vi "UI_Control_System.vi"() -> ()   [LabVIEW 2014]
uses:
  <vilib>/Platform/TimedLoop/XDataNode/timing_clust.ctl
  <vilib>/Platform/TimedLoop/XDataNode/nitl_modes.ctl
  <vilib>/Platform/TimedLoop/XDataNode/wakeup.ctl
  Terminal-Global-SetValues.vi
  <vilib>/Platform/TimedLoop/XDataNode/XDataNode.xnode
  <vilib>/Platform/TimedLoop/XDataNode/XDNodeRunTimeDep.lvlib
panel:
  out "载荷谱修改":bool=TRUE
  in  "载荷谱修改":bool
  in  "停止":bool caption="启动"
  in  "系统执行状态":i32(listbox)
  out "右侧Y位移":sgl[](graph)
  out "右侧X位移":sgl[](graph)
  out "左侧Y位移":sgl[](graph)
  out "左侧X位移":sgl[](graph)
  in  "加载单元查看详细":bool caption="加载单元"
  in  "主轴监测单元查看详细":bool caption="加载单元"
  in  "试验单元查看详细":bool caption="加载单元"
  in  "陪试单元查看详细":bool caption="加载单元"
  in  "实验进度":dbl(slide) scale=0.0..100.0 scale format="%#_g%%"
  out "Data":string caption="当前时间："
  out "轴向位移幅度图":sgl[](graph)
  out "右侧轴心轨迹图":cluster{"电涡流3":sgl[], "电涡流4":sgl[]}(graph)
  out "左侧轴心轨迹图":cluster{"电涡流1":sgl[], "电涡流2":sgl[]}(graph)
  out "转速":sgl
  out "出油温度2":dbl
  out "出油温度1":dbl
  out "试验单元出油温度":dbl
  out "轴承外圈温度":dbl
  out "试验单元摩擦力矩":dbl
  out "声发射频谱图":sgl[](graph)
  out "声发射时间曲线":sgl[](graph)
  out "外壳振动频谱图":dbl(graph)
  out "外壳振动时间曲线":cluster{"加速度2":sgl[]}[](graph)
  out "轴向液压缸加载压力":dbl
  out "径向液压缸加载压力":dbl
  # "轴承测控系统"
  # "检测参数区域"
  # "主轴监测单元"
  # "加载单元"
  # "陪试单元"
  # "实验单元"
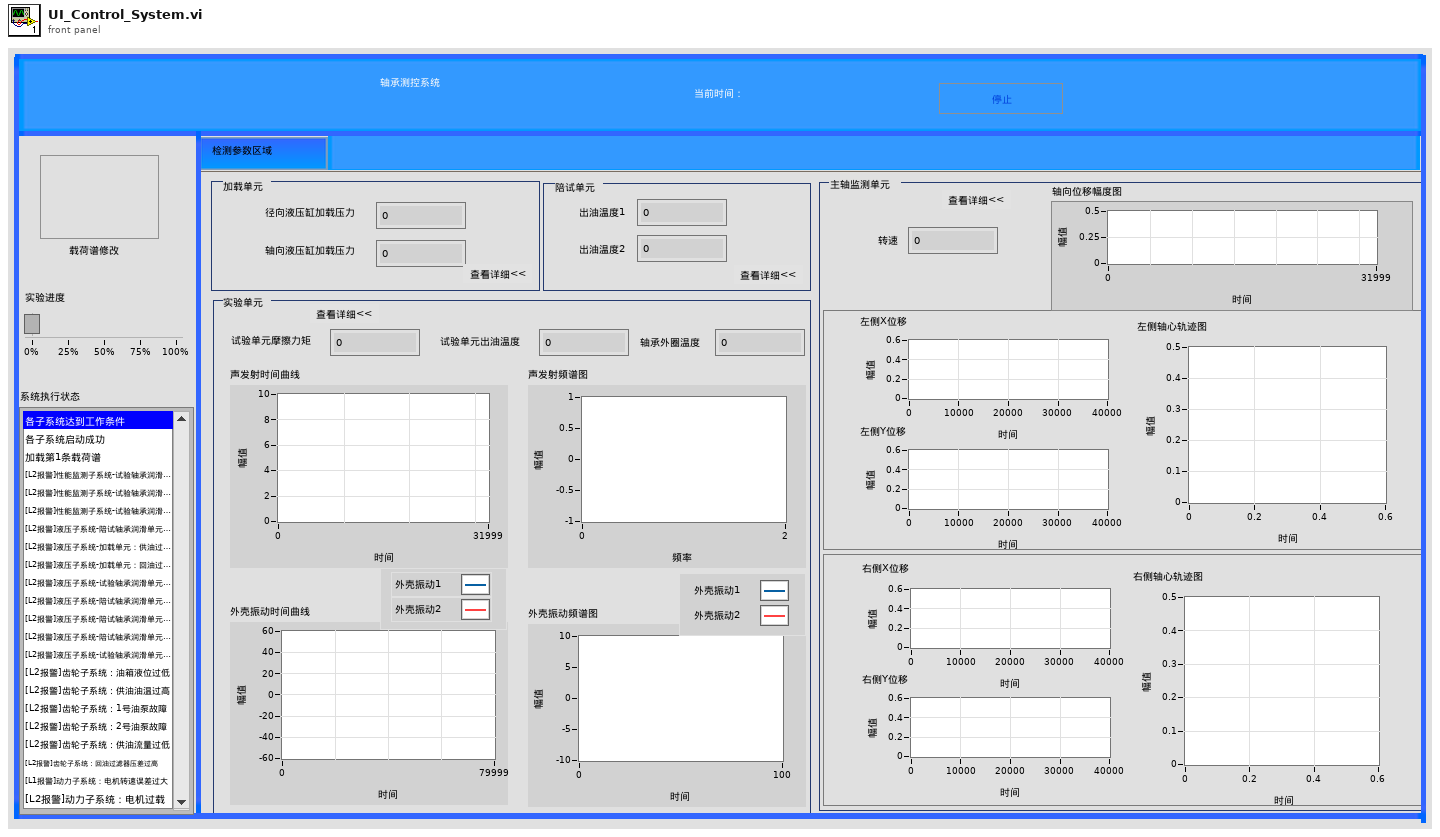
[diagram p1: front panel]
types:
  T1 = typedef "XDNodeRunTimeDep.lvlib/timing_clust.ctl" = cluster{"Expected End [f-1]":u64, "Actual End [f-1]":u64, "Finished Late? [f-1]":bool, "Expected End [i-1]":u64, "Actual End [i-1]":u64, "Finished Late? [i-1]":bool, "Expected Start [i]":u64, "Actual Start [i]":u64, "Expected Start [f]":u64, "Actual Start [f]":u64, "Source Name":string, "Structure Name":string, "Period":i64, "Deadline":i64, "Offset":i64, "Start":i64, "Priority":i32, "Timeout":i32, "Mode":T2, "Wakeup Reason":T3, "Error":errorcluster, "Source Type":string, "Secondary Source Type":string, "Global End Time":u64, "Global Start Time":u64, "Frame Duration":u64, "Iteration Duration":u64, "Assigned CPU":i32, "I/O Scan Engine Mode":u32}
  T2 = typedef "XDNodeRunTimeDep.lvlib/nitl_modes.ctl" = enum32{"No Change", "Process missed periods, maintain original phase", "Discard missed periods, maintain original phase", "Process missed periods, ignore original phase", "Discard missed periods, ignore original phase"}
  T3 = typedef "XDNodeRunTimeDep.lvlib/wakeup.ctl" = enum32{"Normal", "Aborted", "Asynchronous wakeup", "Timing source error", "Timed loop error", "Timeout"}
  T4 = cluster{"润滑油流量":u16, "油箱润滑油液位":u16, "油箱温度":u16, "冷却装置工作状态":u16, "供油压力":u16, "过滤器压差":u16, "油箱液位":u16, "供油油温":u16, "齿轮箱轴承温度":u16, "齿轮箱高速端输出转速":u16, "齿轮子系统状态字":cluster{"加热装置异常报警":bool, "冷却装置异常报警":bool, "油箱液位过低报警":bool, "供油油温过高报警":bool, "循环回路过滤器压差过高报警":bool, "1号油泵故障报警":bool, "2号油泵故障报警":bool, "供油压力过低报警":bool, "供油流量过低报警":bool, "轴承温度异常报警":bool, "油箱液位过高报警":bool, "回油过滤器压差过高报警":bool, "供油过滤器压差过高报警":bool}}
  T5 = cluster{"径向油缸加载压力":u16, "轴向油缸加载压力":u16, "油箱1油液温度":u16, "润滑油温度":u16, "油箱2油液温度":u16, "试验轴承供油压力":u16, "试验轴承供油流量":u16, "陪试轴承供油流量":u16, "陪试轴承供油压力":u16, "陪试轴承供油温度":u16, "液压子系统状态字":cluster{"加载单元":cluster{"供油过滤器堵塞报警":bool, "回油过滤器堵塞报警":bool, "液位过高报警":bool, "液位过低报警":bool}, "试验轴承单元":cluster{"加热装置异常报警":bool, "油箱1液位过高报警":bool, "油箱1液位过低报警":bool, "油箱2液位过高报警":bool, "油箱2液位过低报警":bool, "供油过滤器堵塞报警":bool, "循环回路过滤器堵塞报警":bool, "回油过滤器堵塞报警":bool}, "陪试轴承单元":cluster{"供油过滤器1堵塞报警":bool, "供油过滤器2堵塞报警":bool, "回油过滤器堵塞报警":bool, "油箱液位过高报警":bool, "油箱液位过低报警":bool}}}
  T6 = cluster{"时间":timestamp, "陪试轴承润滑单元出油温度1":sgl[], "陪试轴承润滑单元出油温度2":sgl[], "轴承外圈温度":sgl[], "出油温度":sgl[], "摩擦力1":sgl[], "摩擦力2":sgl[], "径向油缸力":sgl[], "轴向油缸力":sgl[], "转速":sgl[]}
  T7 = cluster{"时间":timestamp, "声发射":sgl[], "电涡流1":sgl[], "电涡流2":sgl[], "电涡流3":sgl[], "电涡流4":sgl[], "电涡流5":sgl[], "加速度1":sgl[], "加速度2":sgl[]}
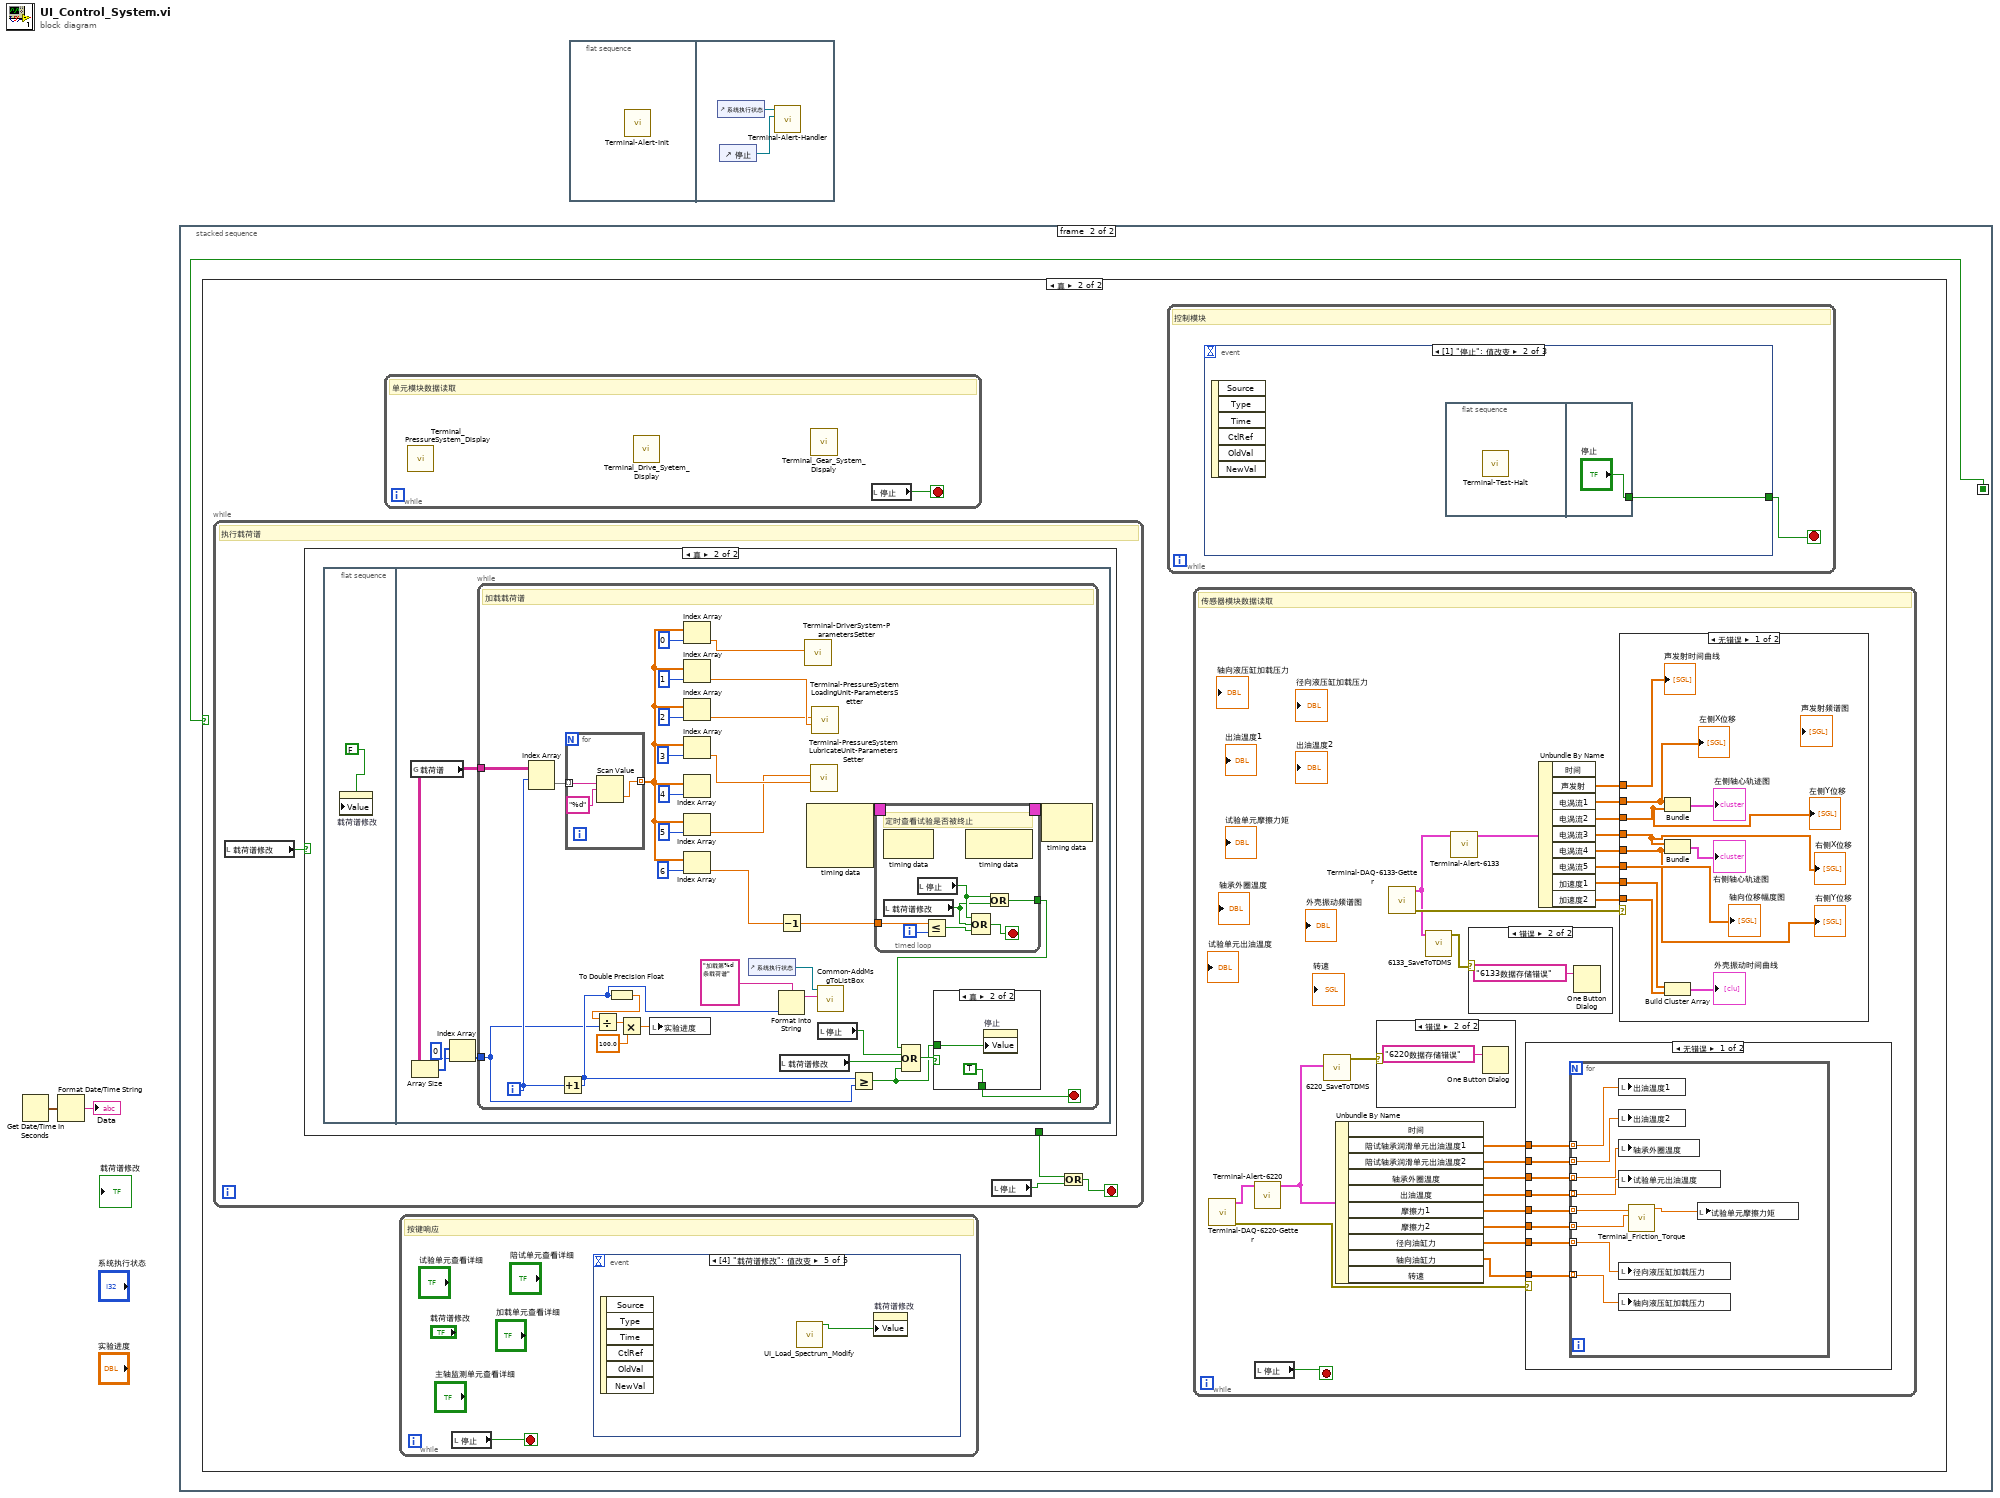
[diagram p0: block diagram]
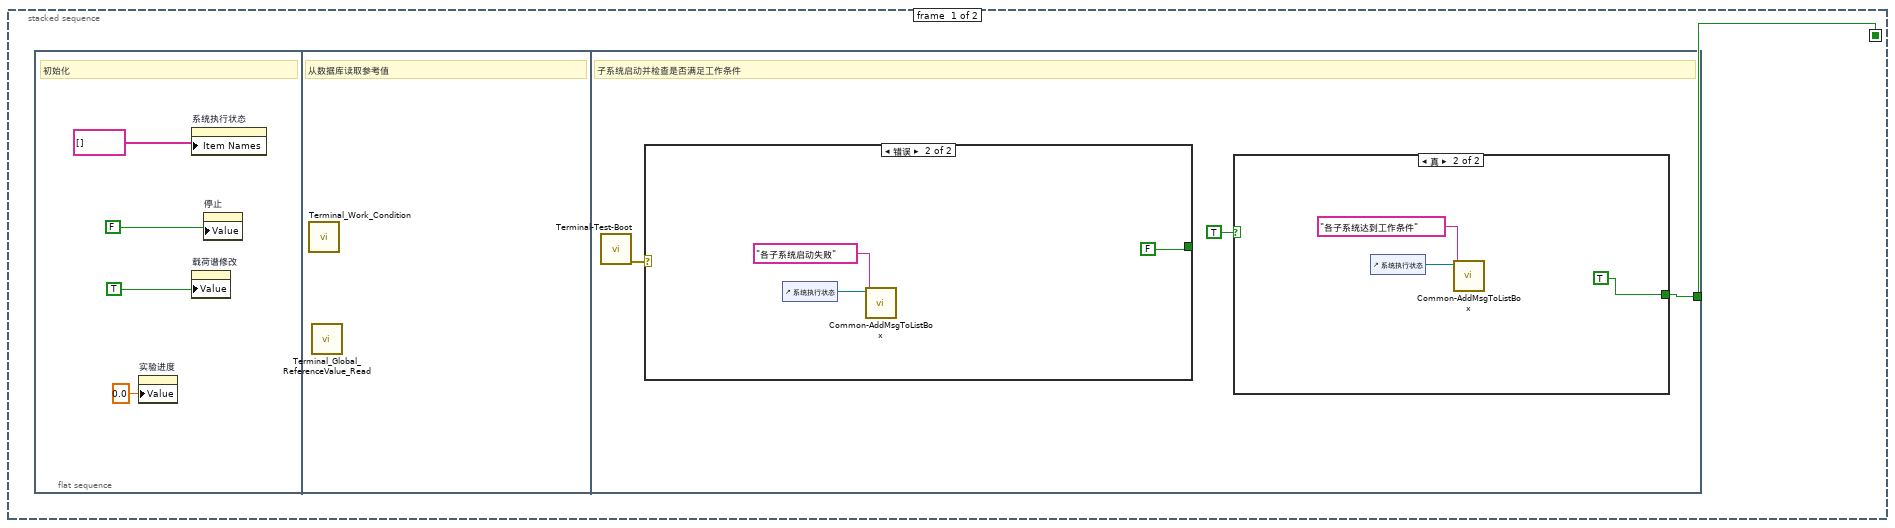
[diagram p2: hidden frame]
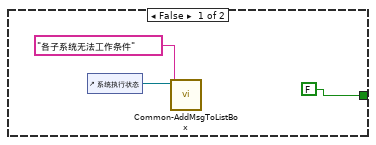
[diagram p3: hidden frame]
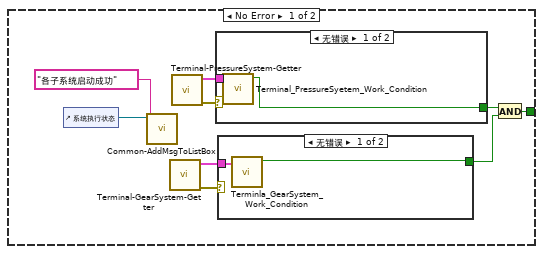
[diagram p4: hidden frame]
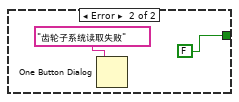
[diagram p5: hidden frame]
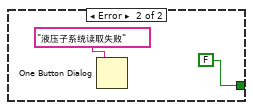
[diagram p6: hidden frame]
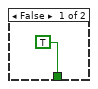
[diagram p8: hidden frame]
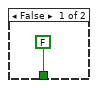
[diagram p9: hidden frame]
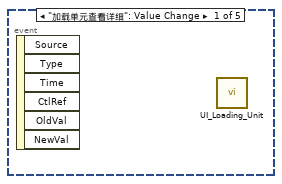
[diagram p10: hidden frame]
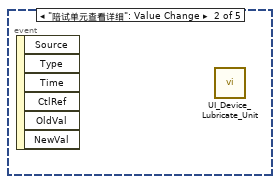
[diagram p11: hidden frame]
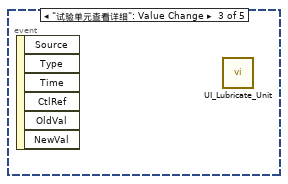
[diagram p12: hidden frame]
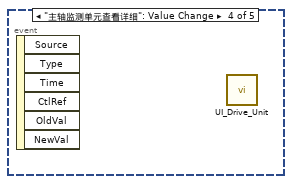
[diagram p13: hidden frame]
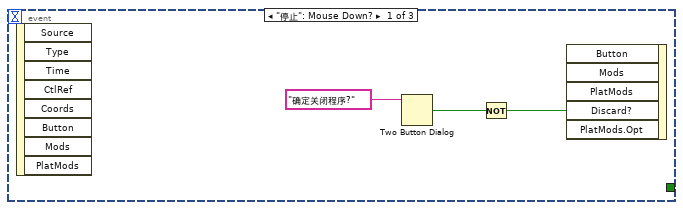
[diagram p18: hidden frame]
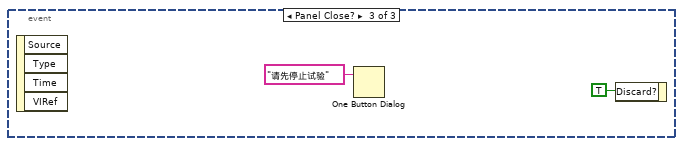
[diagram p19: hidden frame]
diagram:
  n1 = Get Date/Time In Seconds() -> (seconds since 1Jan1904=w1:timestamp)
  n2 = Format Date/Time String(seconds (now)=w1) -> (date/time string=→"Data":string)  [unwired: 2 in]
  n3 = stacked-sequence {
    seq-local: [w3 _] -> [_ w37]
    frame #0 {
      n4 = flat-sequence {
        tunnel: [w8] -> w3
        frame #0 {
          # "初始化"
          n5 = property on="实验进度" class="Slide (严格)"("Value"=0.0 ("实验进度")) -> ()  [unwired: 2 in, 2 out]
          n6 = property on="系统执行状态" class="LstBox (严格)"("Item Names"=string[] [] ("项名")) -> ()  [unwired: 2 in, 2 out]
          n7 = property on="载荷谱修改" class="Bool (严格)"("Value"=TRUE) -> ()  [unwired: 2 in, 2 out]
          n8 = property on="停止" class="Bool (严格)"("Value"=FALSE) -> ()  [unwired: 2 in, 2 out]
        }
        frame #1 {
          # "从数据库读取参考值"
          n9 = call "Terminal_Work_Condition.vi"() -> ()  [unwired: 12 in]
          n10 = call "Terminal_Global_ReferenceValue_Read.vi"() -> ()  [unwired: 12 in]
        }
        frame #2 {
          # "子系统启动并检查是否满足工作条件"
          n11 = call "Terminal-Test-Boot.vi"() -> ("error out"=w10:errorcluster)  [unwired: 11 in]
          n12 = case shown="错误" w10 {
            tunnel: [w21 FALSE] -> _
            frame No Error {
              n13 = control-ref of="系统执行状态"() -> (w17:refnum<vi>)
              n14 = call "Common-AddMsgToListBox.vi"("字符串"="各子系统启动成功", "列表框"=w17) -> ()  [unwired: 10 in]
              n15 = call "Terminal-GearSystem-Getter.vi"() -> ("error out"=w19:errorcluster, "设备信息"=w24:T4)  [unwired: 9 in, 1 out]
              n16 = call "Terminal-PressureSystem-Getter.vi"() -> ("error out"=w20:errorcluster, "设备信息"=w25:T5)  [unwired: 9 in, 1 out]
              n17 = case shown="无错误" w20 {
                tunnel: w25 -> [w31 _]
                tunnel: [w30 FALSE] -> w23
                frame No Error {
                  n18 = call "Terminal_PressureSyetem_Work_Condition.vi"("液压子系统监测参数"=w31) -> ("达到工作条件"=w30:bool)  [unwired: 10 in]
                }
                frame Error {
                  n19 = One Button Dialog(message="液压子系统读取失败" ("消息")) -> ()  [unwired: 1 in, 1 out]
                }
              }
              n20 = case shown="无错误" w19 {
                tunnel: w24 -> [w27 _]
                tunnel: [w26 FALSE] -> w22
                frame No Error {
                  n21 = call "Terminla_GearSystem_Work_Condition.vi"("齿轮子系统监测参数"=w27) -> ("达到工作条件"=w26:bool)  [unwired: 10 in]
                }
                frame Error {
                  n22 = One Button Dialog(message="齿轮子系统读取失败" ("消息")) -> ()  [unwired: 1 in, 1 out]
                }
              }
              n23 = And(x=w23, y=w22) -> (x .and. y?=w21:bool)
            }
            frame Error {
              n24 = control-ref of="系统执行状态"() -> (w34:refnum<vi>)
              n25 = call "Common-AddMsgToListBox.vi"("字符串"="各子系统启动失败", "列表框"=w34) -> ()  [unwired: 10 in]
            }
          }
          n26 = case shown="真" TRUE {
            tunnel: [FALSE TRUE] -> w8
            frame False {
              n27 = control-ref of="系统执行状态"() -> (w13:refnum<vi>)
              n28 = call "Common-AddMsgToListBox.vi"("字符串"="各子系统无法工作条件", "列表框"=w13) -> ()  [unwired: 10 in]
            }
            frame True {
              n29 = control-ref of="系统执行状态"() -> (w16:refnum<vi>)
              n30 = call "Common-AddMsgToListBox.vi"("字符串"="各子系统达到工作条件", "列表框"=w16) -> ()  [unwired: 10 in]
            }
          }
        }
      }
    }
    frame #1 {
      n31 = case shown="真" w37 {
        frame False {
        }
        frame True {
          n32 = while {
            stop <- w39 stop-if-true
            # "执行载荷谱"
            n33 = local read "载荷谱修改"() -> (w41:bool)
            n34 = case shown="真" w41 {
              tunnel: [TRUE _] -> w38
              frame False {
              }
              frame True {
                n35 = flat-sequence {
                  frame #0 {
                    n36 = property on="载荷谱修改" class="Bool (严格)"("Value"=FALSE) -> ()  [unwired: 2 in, 2 out]
                  }
                  frame #1 {
                    n37 = global read "Terminal-Global-SetValues.vi" "载荷谱"() -> (w47:string[][])
                    n38 = Array Size(array=w47) -> (size(s)=w46:i32[])
                    n39 = Index Array(array=w46, index=0 ("索引")) -> (element=w45:i32)
                    n40 = while {
                      tunnel: w47 -> [w66]
                      tunnel: w45 -> [w57]
                      i -> [w65]
                      stop <- w58 stop-if-true
                      # "加载载荷谱"
                      n41 = Index Array(array=w66, index (row)=w65) -> (element=w82:string[])  [unwired: 1 in]
                      n42 = Increment(x=w65) -> (x+1=w59:i32)
                      n43 = for {
                        tunnel: w82 -> [w99] mode=indexing
                        tunnel: [w97] -> w81 mode=indexing
                        n44 = Scan Value(string=w99, format string="%d" ("格式字符串")) -> (value=w97:dbl)  [unwired: 1 in, 1 out]
                      }
                      n45 = To Double Precision Float(number=w59) -> (double precision float=w64:dbl)
                      n46 = Divide(x=w64, y=w57) -> (x/y=w62:dbl)
                      n47 = Multiply(x=w62, y=100.0) -> (x*y=w60:dbl)
                      n48 = local write "实验进度"(w60) -> ()
                      n49 = Index Array(array=w81, index=0 ("索引")) -> (element=w71:dbl)
                      n50 = Index Array(array=w81, index=1 ("索引")) -> (element=w70:dbl)
                      n51 = Index Array(array=w81, index=2 ("索引")) -> (element=w69:dbl)
                      n52 = Index Array(array=w81, index=3 ("索引")) -> (element=w68:dbl)
                      n53 = Index Array(array=w81, index=4 ("索引")) -> ()  [unwired: 1 out]
                      n54 = Index Array(array=w81, index=5 ("索引")) -> (element=w67:dbl)
                      n55 = Index Array(array=w81, index=6 ("索引")) -> (element=w54:dbl)
                      n56 = control-ref of="系统执行状态"() -> (w73:refnum<vi>)
                      n57 = Decrement(x=w54) -> (x-1=w53:dbl)
                      n58 = Format Into String(format string="加载第%d条载荷谱" ("字符串"), w59) -> (resulting string=w72:string)  [unwired: 2 in, 1 out]
                      n59 = local read "载荷谱修改"() -> (w50:bool)
                      n60 = call "Terminal-DriverSystem-ParametersSetter.vi"("转速"=w71) -> ()  [unwired: 10 in, 1 out]
                      n61 = node-c288() -> (w56:T1)  [unwired: 3 in]
                      n62 = call "Terminal-PressureSystemLubricateUnit-ParametersSetter.vi"("供油润滑温度T"=w68, "供油流量L"=w67) -> ()  [unwired: 9 in, 1 out]
                      n63 = call "Terminal-PressureSystemLoadingUnit-ParametersSetter.vi"("轴向载荷F2"=w70, "径向载荷F1"=w69) -> ()  [unwired: 9 in, 1 out]
                      n64 = call "Common-AddMsgToListBox.vi"("字符串"=w72, "列表框"=w73) -> ()  [unwired: 10 in]
                      n65 = local read "停止"() -> (w51:bool)
                      n66 = Greater Or Equal?(x=w59, y=w57) -> (x >= y?=w49:bool)
                      n67 = timed-loop {
                        timing: w56 -> [_]
                        timing-out: [_] -> w55
                        tunnel: w53 -> [w89]
                        tunnel: [w83] -> w48
                        i -> [w88]
                        stop <- w87 stop-if-true
                        # "定时查看试验是否被终止"
                        n68 = node-c288() -> ()  [unwired: 1 in, 1 out]
                        n69 = local read "载荷谱修改"() -> (w84:bool)
                        n70 = local read "停止"() -> (w85:bool)
                        n71 = Less Or Equal?(x=w89, y=w88) -> (x <= y?=w86:bool)
                        n72 = node-c288() -> ()  [unwired: 1 in, 1 out]
                        n73 = Compound Arithmetic op=OR(w85, w84, w86) -> (w87:bool)
                        n74 = Or(x=w85, y=w84) -> (x .or. y?=w83:bool)
                      }
                      n75 = Compound Arithmetic op=OR(w48, w51, w50, w49) -> (w52:bool)
                      n76 = case shown="真" w52 {
                        tunnel: [FALSE ("停止") TRUE ("停止")] -> w58
                        tunnel: w49 -> [_ w95]
                        frame False {
                        }
                        frame True {
                          n77 = property on="停止" class="Bool (严格)"("Value"=w95) -> ()  [unwired: 2 in, 2 out]
                        }
                      }
                      n78 = node-c288(w55) -> ()  [unwired: 1 out]
                    }
                  }
                }
              }
            }
            n79 = local read "停止"() -> (w40:bool)
            n80 = Or(x=w38, y=w40) -> (x .or. y?=w39:bool)
          }
          n81 = while {
            stop <- w102 stop-if-true
            # "单元模块数据读取"
            n82 = call "Terminal_PressureSystem_Display.vi"() -> ()  [unwired: 12 in]
            n83 = call "Terminal_Drive_Syetem_Display.vi"() -> ()  [unwired: 12 in]
            n84 = call "Terminal_Gear_System_Dispaly.vi"() -> ()  [unwired: 12 in]
            n85 = local read "停止"() -> (w102:bool)
          }
          n86 = while {
            stop <- w100 stop-if-true
            # "按键响应"
            n87 = local read "停止"() -> (w100:bool)
            n88 = event shown="[4] \"载荷谱修改\": 值改变" {
              selector: _ -> [_ _ _ _ _]
              dyn-events: _ -> [_ _ _ _ _]
              timeout: _ -> [_ _ _ _ _]
              event "加载单元查看详细": Value Change {
                n89 = event-data() -> ()  [unwired: 1 in, 6 out]
                n90 = call "UI_Loading_Unit.vi"() -> ()  [unwired: 12 in]
              }
              event "陪试单元查看详细": Value Change {
                n91 = event-data() -> ()  [unwired: 1 in, 6 out]
                n92 = call "UI_Device_Lubricate_Unit.vi"() -> ()  [unwired: 12 in]
              }
              event "试验单元查看详细": Value Change {
                n93 = event-data() -> ()  [unwired: 1 in, 6 out]
                n94 = call "UI_Lubricate_Unit.vi"() -> ()  [unwired: 12 in]
              }
              event "主轴监测单元查看详细": Value Change {
                n95 = event-data() -> ()  [unwired: 1 in, 6 out]
                n96 = call "UI_Drive_Unit.vi"() -> ()  [unwired: 12 in]
              }
              event "载荷谱修改": Value Change {
                n97 = event-data() -> ()  [unwired: 1 in, 6 out]
                n98 = call "UI_Load_Spectrum_Modify.vi"() -> ("载荷谱修改"=w101:bool)  [unwired: 11 in]
                n99 = property on="载荷谱修改" class="Bool (严格)"("Value"=w101) -> ()  [unwired: 2 in, 2 out]
              }
            }
          }
          n100 = while {
            stop <- w158 stop-if-true
            # "控制模块"
            n101 = event shown="[1] \"停止\": 值改变" {
              selector: _ -> [_ _ _]
              dyn-events: _ -> [_ _ _]
              timeout: _ -> [_ _ _]
              tunnel: [_ w162 _] -> w158
              event "停止": Mouse Down? {
                n102 = event-data() -> ()  [unwired: 1 in, 8 out]
                n103 = Two Button Dialog(message="确定关闭程序?" ("消息")) -> (T button?=w160:bool)  [unwired: 2 in]
                n104 = Not(x=w160) -> (.not. x?=w159:bool)
                n105 = event-data("Discard?"=w159) -> ()  [unwired: 5 in, 1 out]
              }
              event "停止": Value Change {
                n106 = event-data() -> ()  [unwired: 1 in, 6 out]
                n107 = flat-sequence {
                  tunnel: ["停止"] -> w162
                  frame #0 {
                    n108 = call "Terminal-Test-Halt.vi"() -> ()  [unwired: 11 in, 1 out]
                  }
                  frame #1 {
                  }
                }
              }
              event Panel Close? {
                n109 = event-data() -> ()  [unwired: 1 in, 4 out]
                n110 = One Button Dialog(message="请先停止试验" ("消息")) -> ()  [unwired: 1 in, 1 out]
                n111 = event-data("Discard?"=TRUE ("放弃？")) -> ()  [unwired: 1 in, 1 out]
              }
            }
          }
          n112 = while {
            stop <- w109 stop-if-true
            # "传感器模块数据读取"
            n113 = call "Terminal-DAQ-6220-Getter.vi"() -> ("error out"=w119:errorcluster, "6220"=w104:T6)  [unwired: 10 in]
            n114 = call "Terminal-Alert-6220.vi"("6220"=w104) -> ("6220输出"=w103:T6)  [unwired: 10 in]
            n115 = local read "停止"() -> (w109:bool)
            n116 = call "6220_SaveToTDMS.vi"("数据"=w103) -> ("错误输出"=w108:errorcluster)  [unwired: 10 in]
            n117 = Unbundle By Name(w103) -> ("陪试轴承润滑单元出油温度1"=w117:sgl[], "陪试轴承润滑单元出油温度2"=w116:sgl[], "轴承外圈温度"=w115:sgl[], "出油温度"=w114:sgl[], "摩擦力1"=w113:sgl[], "摩擦力2"=w112:sgl[], "径向油缸力"=w118:sgl[], "轴向油缸力"=w111:sgl[])  [unwired: 2 out]
            n118 = case shown="错误" w108 {
              frame No Error {
              }
              frame Error {
                n119 = One Button Dialog(message="6220数据存储错误" ("消息")) -> ()  [unwired: 1 in, 1 out]
              }
            }
            n120 = call "Terminal-DAQ-6133-Getter.vi"() -> ("error out"=w127:errorcluster, "6133"=w106:T7)  [unwired: 10 in]
            n121 = call "6133_SaveToTDMS.vi"("数据"=w106) -> ("错误输出"=w107:errorcluster)  [unwired: 10 in]
            n122 = call "Terminal-Alert-6133.vi"("6133"=w106) -> ("6133输出"=w105:T7)  [unwired: 10 in]
            n123 = case shown="错误" w107 {
              frame No Error {
              }
              frame Error {
                n124 = One Button Dialog(message="6133数据存储错误" ("消息")) -> ()  [unwired: 1 in, 1 out]
              }
            }
            n125 = case shown="无错误" w119 {
              tunnel: w118 -> [w137 _]
              tunnel: w117 -> [w136 _]
              tunnel: w116 -> [w135 _]
              tunnel: w115 -> [w134 _]
              tunnel: w114 -> [w133 _]
              tunnel: w113 -> [w132 _]
              tunnel: w112 -> [w131 _]
              tunnel: w111 -> [w130 _]
              frame No Error {
                n126 = for {
                  tunnel: w137 -> [w146] mode=indexing
                  tunnel: w136 -> [w145] mode=indexing
                  tunnel: w135 -> [w144] mode=indexing
                  tunnel: w134 -> [w143] mode=indexing
                  tunnel: w133 -> [w142] mode=indexing
                  tunnel: w132 -> [w141] mode=indexing
                  tunnel: w131 -> [w140] mode=indexing
                  tunnel: w130 -> [w138] mode=indexing
                  n127 = local write "出油温度1"(w145) -> ()
                  n128 = local write "出油温度2"(w144) -> ()
                  n129 = local write "轴承外圈温度"(w143) -> ()
                  n130 = local write "试验单元出油温度"(w142) -> ()
                  n131 = local write "径向液压缸加载压力"(w146) -> ()
                  n132 = local write "轴向液压缸加载压力"(w138) -> ()
                  n133 = call "Terminal_Friction_Torque.vi"("摩擦力FR"=w140, "摩擦力FL"=w141) -> ("摩擦力矩"=w139:dbl)  [unwired: 9 in]
                  n134 = local write "试验单元摩擦力矩"(w139) -> ()
                }
              }
              frame Error {
              }
            }
            n135 = Unbundle By Name(w105) -> ("声发射"=w124:sgl[], "电涡流1"=w126:sgl[], "电涡流2"=w125:sgl[], "电涡流3"=w123:sgl[], "电涡流4"=w122:sgl[], "电涡流5"=w110:sgl[], "加速度1"=w121:sgl[], "加速度2"=w120:sgl[])  [unwired: 1 out]
            n136 = case shown="无错误" w127 {
              tunnel: w124 -> [w152 _]
              tunnel: w126 -> [w150 _]
              tunnel: w125 -> [w149 _]
              tunnel: w121 -> [w155 _]
              tunnel: w120 -> [w153 _]
              tunnel: w123 -> [w148 _]
              tunnel: w122 -> [w147 _]
              tunnel: w110 -> [w151 _]
              frame No Error {
                n137 = Bundle("电涡流1"=w150, "电涡流2"=w149) -> (→"左侧轴心轨迹图":cluster{"电涡流1":sgl[], "电涡流2":sgl[]})  [unwired: 1 in]
                n138 = Bundle("电涡流3"=w148, "电涡流4"=w147) -> (→"右侧轴心轨迹图":cluster{"电涡流3":sgl[], "电涡流4":sgl[]})  [unwired: 1 in]
                n139 = Build Cluster Array(w155, w153) -> (→"外壳振动时间曲线":cluster{"加速度2":sgl[]}[])
                "轴向位移幅度图" <- w151
                "声发射时间曲线" <- w152
                "左侧X位移" <- w150
                "左侧Y位移" <- w149
                "右侧Y位移" <- w147
                "右侧X位移" <- w148
              }
              frame Error {
              }
            }
          }
        }
      }
    }
  }
  n140 = flat-sequence {
    frame #0 {
      n141 = call "Terminal-Alert-Init.vi"() -> ()  [unwired: 12 in]
    }
    frame #1 {
      n142 = control-ref of="系统执行状态"() -> (w167:refnum<vi>)
      n143 = control-ref of="停止"() -> (w166:refnum<vi>)
      n144 = call "Terminal-Alert-Handler.vi"("开关"=w166, "列表框"=w167) -> ()  [unwired: 10 in]
    }
  }
